vi "TCP Safe Read.vi"(8 "error in (no error)":errorcluster, 9 "timeout ms (25000)":i32, 10 "bytes to read":i32, 11 "TCP Network Connection in":refnum<k5>) -> (0 "error out":errorcluster, 2 "String":string, 3 "TCP Network Connection out":refnum<k5>)   [LabVIEW 2020, in "CSM-TCP-Router.lvlib"]
uses:
  CSM-TCP-Router.lvlib
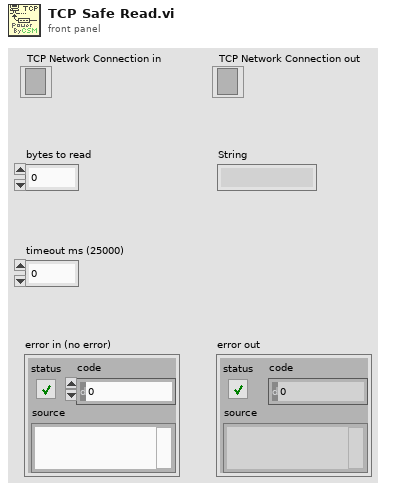
[diagram p1: front panel]
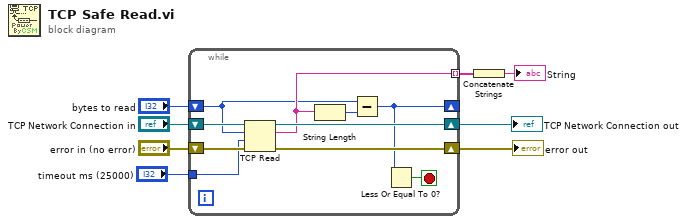
[diagram p0: block diagram]
diagram:
  n1 = while {
    tunnel: [w14] -> w6 mode=indexing
    shift-right: [w16] -> w4
    shift-left: "TCP Network Connection in" -> [w18]
    shift-right: [w15] -> w7
    shift-left: "error in (no error)" -> [w17]
    shift-right: [w11] -> _
    shift-left: "bytes to read" -> [w12]
    tunnel: "timeout ms (25000)" -> [w9]
    stop <- w10 stop-if-true
    n2 = TCP Read(connection ID=w18, bytes to read=w12, error in (no error)=w17, 9:w9) -> (connection ID out=w16:refnum<k5>, data out=w14:string, error out=w15:errorcluster)  [unwired: 1 in]
    n3 = String Length(string=w14) -> (length=w13:i32)
    n4 = Subtract(x=w12, y=w13) -> (x-y=w11:i32)
    n5 = Less Or Equal To 0?(x=w11) -> (x <= 0?=w10:bool)
  }
  "error out" <- w7
  "TCP Network Connection out" <- w4
  n6 = Concatenate Strings(w6) -> (→"String":string)
